vi "Load State.vi"(8 "error in (no error)":errorcluster, 10 "instance vi ref":refnum<vi>, 11 "vi ref":refnum<vi>) -> (0 "error out":errorcluster, 1 "State":variant, 2 "Tag Found?":bool, 3 "vi ref out":refnum<vi>)   [LabVIEW 2021]
panel:
  out "instance vi ref out":refnum<vi>
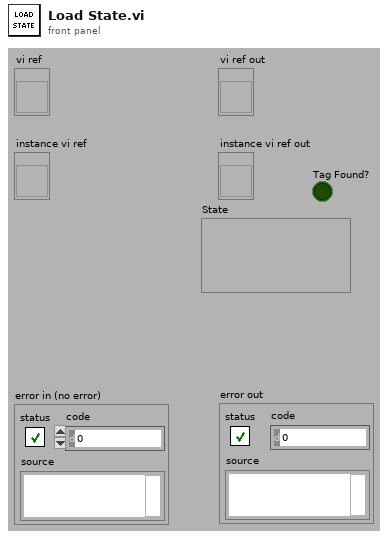
[diagram p1: front panel]
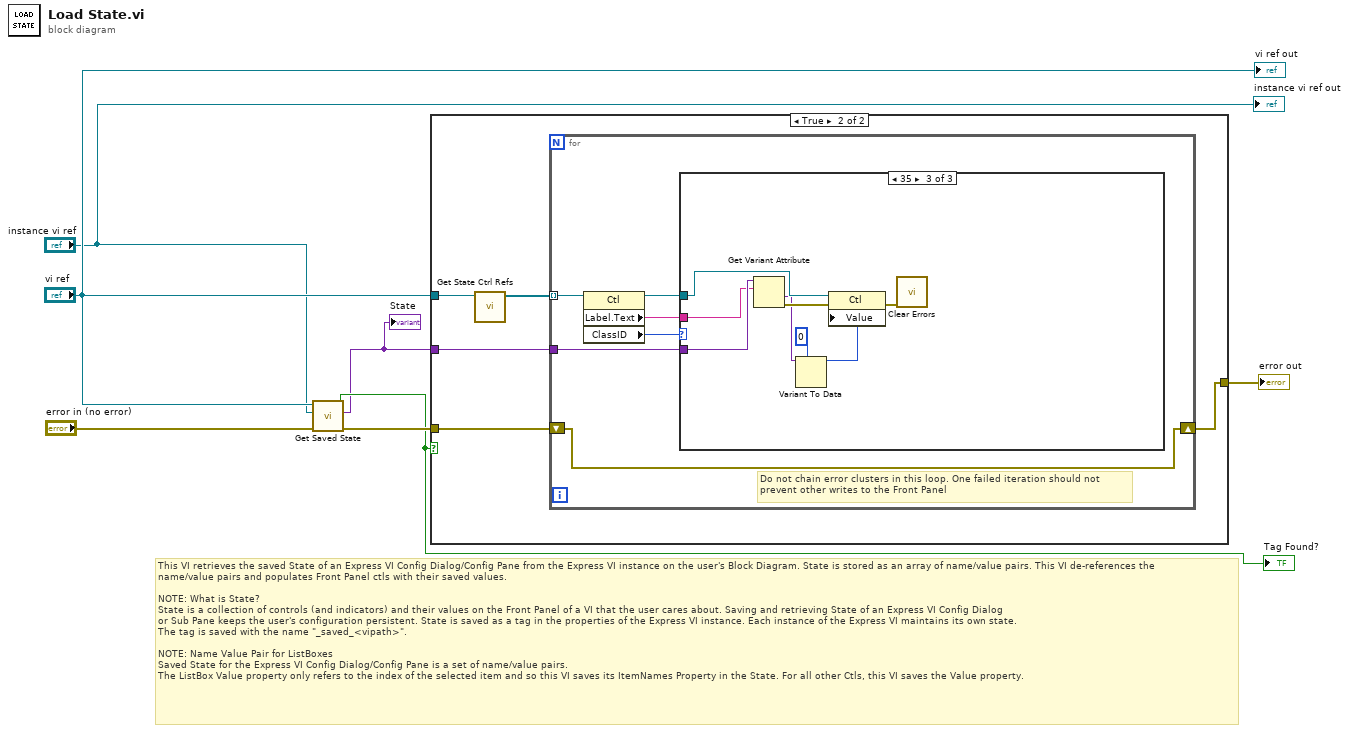
[diagram p0: block diagram]
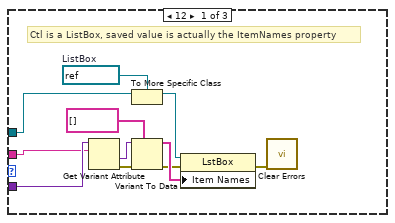
[diagram p3: hidden frame]
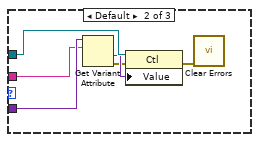
[diagram p4: hidden frame]
diagram:
  # "This VI retrieves the saved State of an Express VI Config Dialog/Config Pane from the Express VI instance on the user's Block Diagram. State is stored as an array of name/value pairs. This VI de-references the \nname/value pairs and populates Front Panel ctls with their saved values. \n\nNOTE: What is State?\nState is a collection of controls (and indicators) and their values on the Front Panel of a VI that the user cares about. Saving and retrieving State of an Express VI Config Dialog \nor Sub Pane keeps the user's configuration persistent. State is saved as a tag in the properties of the Express VI instance. Each instance of the Express VI maintains its own state. \nThe tag is saved with the name \"_saved_<vipath>\". \n\nNOTE: Name Value Pair for ListBoxes \nSaved State for the Express VI Config Dialog/Config Pane is a set of name/value pairs.\nThe ListBox Value property only refers to the index of the selected item and so this VI saves its ItemNames Property in the State. For all other Ctls, this VI saves the Value property."
  n1 = call <vilib>:"Get Saved State.vi"("error in (no error)"="error in (no error)", "instance vi ref"="instance vi ref", "vi ref"="vi ref") -> ("error out"=w5:errorcluster, "State"=w1:variant, "Tag Found"=w4:bool)  [unwired: 6 in]
  "Tag Found?" <- w4
  "State" <- w1
  n2 = case shown="True" w4 {
    tunnel: [w8 w11] -> w7
    tunnel: w5 -> [w8 w10]
    tunnel: "vi ref" -> [_ w12]
    tunnel: w1 -> [_ w9]
    frame False {
    }
    frame True {
      n3 = call <vilib>:"Get State Ctrl Refs.vi"("vi ref"=w12) -> ("All Controls[]"=w13:refnum<vi>[])  [unwired: 9 in, 1 out]
      n4 = for {
        tunnel: w13 -> [w17] mode=indexing
        shift-right: [w15] -> w11
        shift-left: w10 -> [w15]
        tunnel: w9 -> [w14]
        # "Do not chain error clusters in this loop. One failed iteration should not \nprevent other writes to the Front Panel"
        n5 = property class="Ctl"(reference=w17) -> (reference out=w19:refnum<vi>, "Label.Text"=w18:string, "ClassID"=w16:u32)  [unwired: 1 in, 1 out]
        n6 = case shown="35" w16 {
          tunnel: w18 -> [w25 w35 w43]
          tunnel: w19 -> [w20 w34 w42]
          tunnel: w14 -> [w26 w36 w44]
          frame 12 {
            w30 = refnum<vi> refnum  # ListBox
            # "Ctl is a ListBox, saved value is actually the ItemNames property"
            n7 = Get Variant Attribute(Variant=w26, name=w25) -> (value=w24:variant, error out=w23:errorcluster)  [unwired: 2 in, 2 out]
            n8 = To More Specific Class(target class=w30, reference=w20) -> (specific class reference=w29:refnum<vi>)  [unwired: 1 in, 1 out]
            n9 = Variant To Data(error in=w23, type=string[] [] ("Item Names"), Variant=w24) -> (data=w27:string[], error out=w22:errorcluster)
            n10 = property class="LstBox"(reference=w29, error in=w22, "Item Names"=w27) -> (error out=w21:errorcluster)  [unwired: 1 out]
            n11 = call <vilib>:"Clear Errors.vi"("error in (no error)"=w21) -> ()  [unwired: 5 in, 2 out]
          }
          frame Default {
            n12 = Get Variant Attribute(Variant=w36, name=w35) -> (value=w33:variant, error out=w32:errorcluster)  [unwired: 2 in, 2 out]
            n13 = property class="Ctl"(reference=w34, error in=w32, "Value"=w33) -> (error out=w31:errorcluster)  [unwired: 1 out]
            n14 = call <vilib>:"Clear Errors.vi"("error in (no error)"=w31) -> ()  [unwired: 5 in, 2 out]
          }
          frame 35 {
            n15 = Get Variant Attribute(Variant=w44, name=w43) -> (value=w39:variant, error out=w41:errorcluster)  [unwired: 2 in, 2 out]
            n16 = Variant To Data(type=u8 0, Variant=w39) -> (data=w37:u8)  [unwired: 1 in, 1 out]
            n17 = property class="Ctl"(reference=w42, error in=w41, "Value"=w37) -> (error out=w40:errorcluster)  [unwired: 1 out]
            n18 = call <vilib>:"Clear Errors.vi"("error in (no error)"=w40) -> ()  [unwired: 5 in, 2 out]
          }
        }
      }
    }
  }
  "error out" <- w7
  "instance vi ref out" <- "instance vi ref"
  "vi ref out" <- "vi ref"
